vi "Run_block.vi"(7 "Oversample":i16, 8 "error in (no error)":errorcluster, 9 "Timebase":i16, 10 "no_of_samples":i16, 11 "Handle":i16) -> (0 "error out":errorcluster, 3 "return type":i16)   [LabVIEW 2023]
uses:
  ps2000.dll
panel:
  in  "*time_indisposed_ms":i16
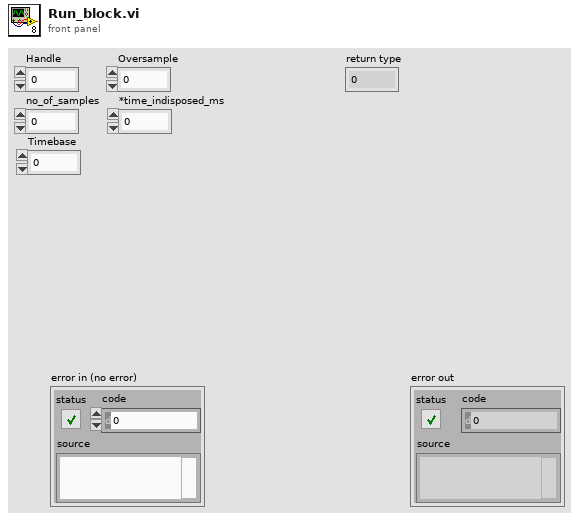
[diagram p1: front panel]
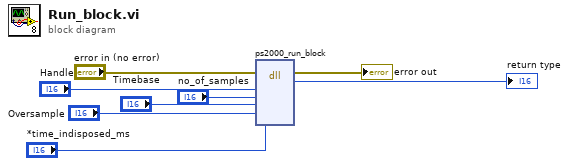
[diagram p0: block diagram]
diagram:
  n1 = dll-call lib="C:/Users/cesar/Desktop/Ps2000 libreria/PS2000.dll" fn="ps2000_run_block"(error in="error in (no error)", "handle"="Handle", "no_of_samples"="no_of_samples", "timebase"="Timebase", "oversample"="Oversample", "*time_indisposed_ms"="*time_indisposed_ms") -> (error out=→"error out":errorcluster, "return type"=→"return type":i16)  [unwired: 7 in, 1 out]
